vi "hexStringToByteData.vi"(10 "数据输入 2":string) -> (1 "字节数":i32, 2 "CANFD_data":T1)   [LabVIEW 2018]
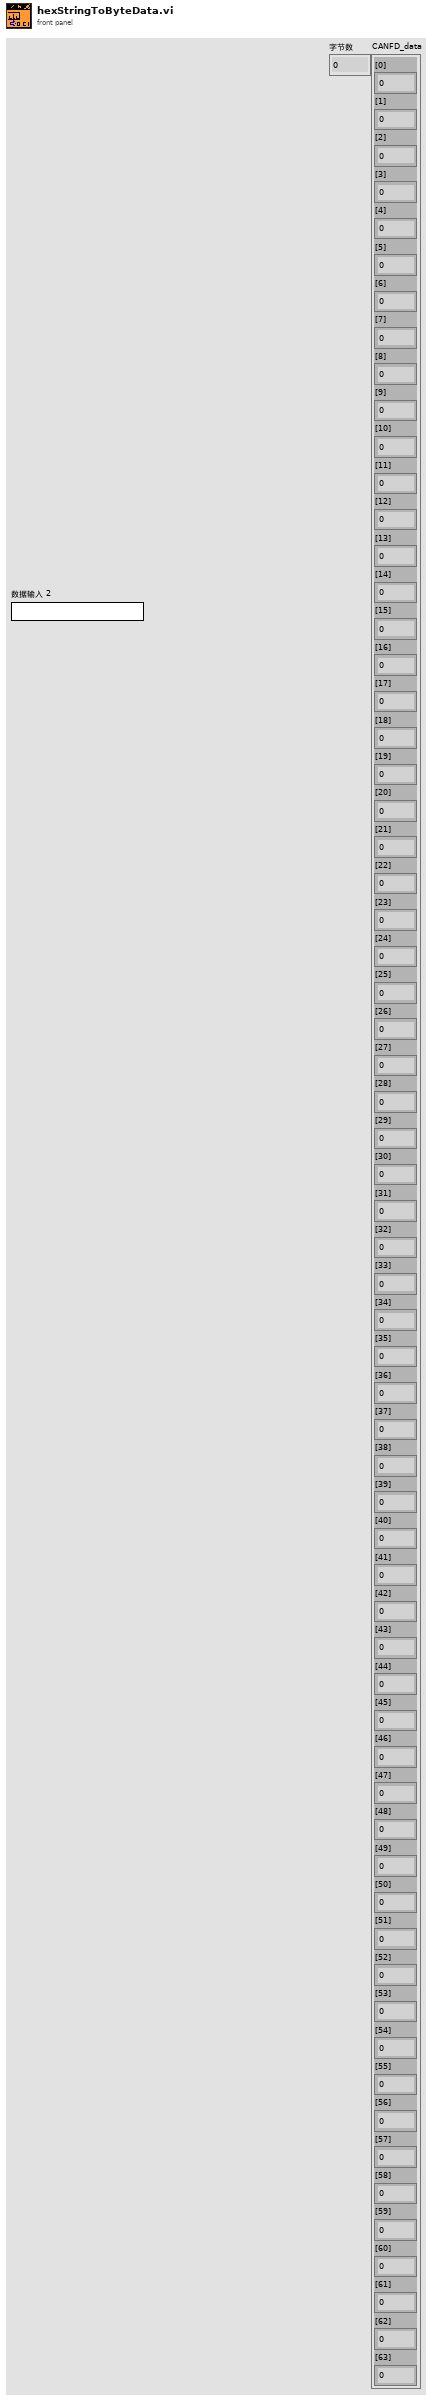
[diagram p1: front panel]
types:
  T1 = cluster{"[0]":u32, "[1]":u32, "[2]":u32, "[3]":u32, "[4]":u32, "[5]":u32, "[6]":u32, "[7]":u32, "[8]":u32, "[9]":u32, "[10]":u32, "[11]":u32, "[12]":u32, "[13]":u32, "[14]":u32, "[15]":u32, "[16]":u32, "[17]":u32, "[18]":u32, "[19]":u32, "[20]":u32, "[21]":u32, "[22]":u32, "[23]":u32, "[24]":u32, "[25]":u32, "[26]":u32, "[27]":u32, "[28]":u32, "[29]":u32, "[30]":u32, "[31]":u32, "[32]":u32, "[33]":u32, "[34]":u32, "[35]":u32, "[36]":u32, "[37]":u32, "[38]":u32, "[39]":u32, "[40]":u32, "[41]":u32, "[42]":u32, "[43]":u32, "[44]":u32, "[45]":u32, "[46]":u32, "[47]":u32, "[48]":u32, "[49]":u32, "[50]":u32, "[51]":u32, "[52]":u32, "[53]":u32, "[54]":u32, "[55]":u32, "[56]":u32, "[57]":u32, "[58]":u32, "[59]":u32, "[60]":u32, "[61]":u32, "[62]":u32, "[63]":u32}
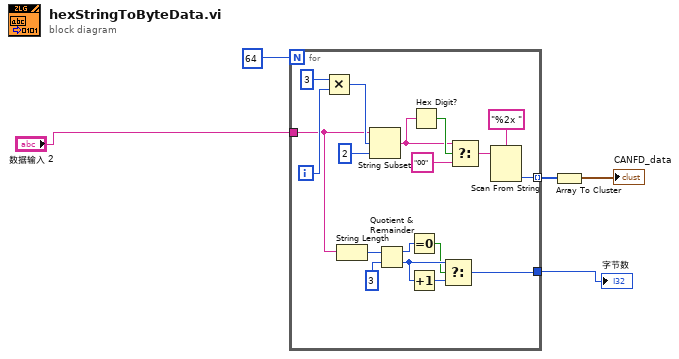
[diagram p0: block diagram]
diagram:
  n1 = for {
    N: 64 -> [_]
    tunnel: "数据输入 2" -> [w8]
    tunnel: [w19] -> w5 mode=indexing
    tunnel: [w6] -> w3
    i -> [w14]
    n2 = Multiply(x=3, y=w14) -> (x*y=w22:i32)
    n3 = String Length(string=w8) -> (length=w13:i32)
    n4 = String Subset(string=w8, offset (0)=w22, length (rest)=2 ("length (rest)")) -> (substring=w16:string)
    n5 = Quotient & Remainder(x=w13, y=3) -> (x-y*floor(x/y)=w11:i32, floor(x/y)=w9:i32)
    n6 = Equal To 0?(x=w11) -> (x = 0?=w7:bool)
    n7 = Increment(x=w9) -> (x+1=w10:i32)
    n8 = Hex Digit?(1:w16) -> (0:w17:bool)
    n9 = Select(t=w9, s=w7, f=w10) -> (s? t:f=w6:i32)
    n10 = Select(t=w16, s=w17, f="00" ("t")) -> (s? t:f=w18:string)
    n11 = Scan From String(format string="%2x ", input string=w18) -> (output 1=w19:u32)  [unwired: 2 in, 4 out]
  }
  "字节数" <- w3
  n12 = Array To Cluster(array=w5) -> (cluster=→"CANFD_data":T1)
